vi "Response - Set Status Code.vi"() -> (3 "Unit Test Framework Results":T1)   [LabVIEW 2023, in "Response.lvclass"]
doc: "Use this template to create a user-defined test VI. Define your test requirements and wire the results to the <b>Result (Test)</b> control. Do not modify the <b>Unit Test Framework Results</b> indicator."
uses:
  Response.lvclass
  <vilib>/utf/common/utf_test_comparison_operators.ctl
  <vilib>/utf/NI_UnitTestFramework.lvlib
  <vilib>/utf/common/utf_test_result.ctl
  <vilib>/utf/common/utf_test_result_failure.ctl
  <vilib>/utf/common/utf_test_result_troll.ctl
  <vilib>/utf/common/utf_vi_tag.ctl
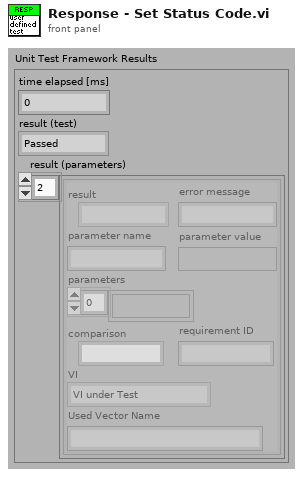
[diagram p1: front panel]
types:
  T1 = typedef "NI_UnitTestFramework.lvlib/utf_test_result_troll.ctl" = cluster{"time elapsed [ms]":u32, "result (test)":T2, "result (parameters)":T3[]}
  T2 = typedef "NI_UnitTestFramework.lvlib/utf_test_result.ctl" = enum16{"Passed", "Failed", "Error", "Skipped", "Not Processed"}
  T3 = typedef "NI_UnitTestFramework.lvlib/utf_test_result_failure.ctl" = cluster{"result":T2, "error message":string, "parameter name":string, "parameter value":variant, "parameters":variant[], "comparison":T4, "requirement ID":string, "VI":T5, "Used Vector Name":string}
  T4 = typedef "NI_UnitTestFramework.lvlib/utf_test_comparison_operators.ctl" = enum16{"=", "!=", ">", ">=", "<", "<=", "range", "symmetric tolerance", "asymmetric tolerance", "string contains", "string not contain", "array size", "string length", "array range", "by element", "array range (limit array)", "user-defined", "array contains", "array not contain", "vector length", "= (elm)", "!= (elm)", "= (case insensitive)", "!= (case insensitive)"}
  T5 = typedef "NI_UnitTestFramework.lvlib/utf_vi_tag.ctl" = enum16{"Setup VI", "VI under Test", "Teardown VI"}
  T6 = typedef "Response.lvclass/Standard Response Messages.ctl" = u16
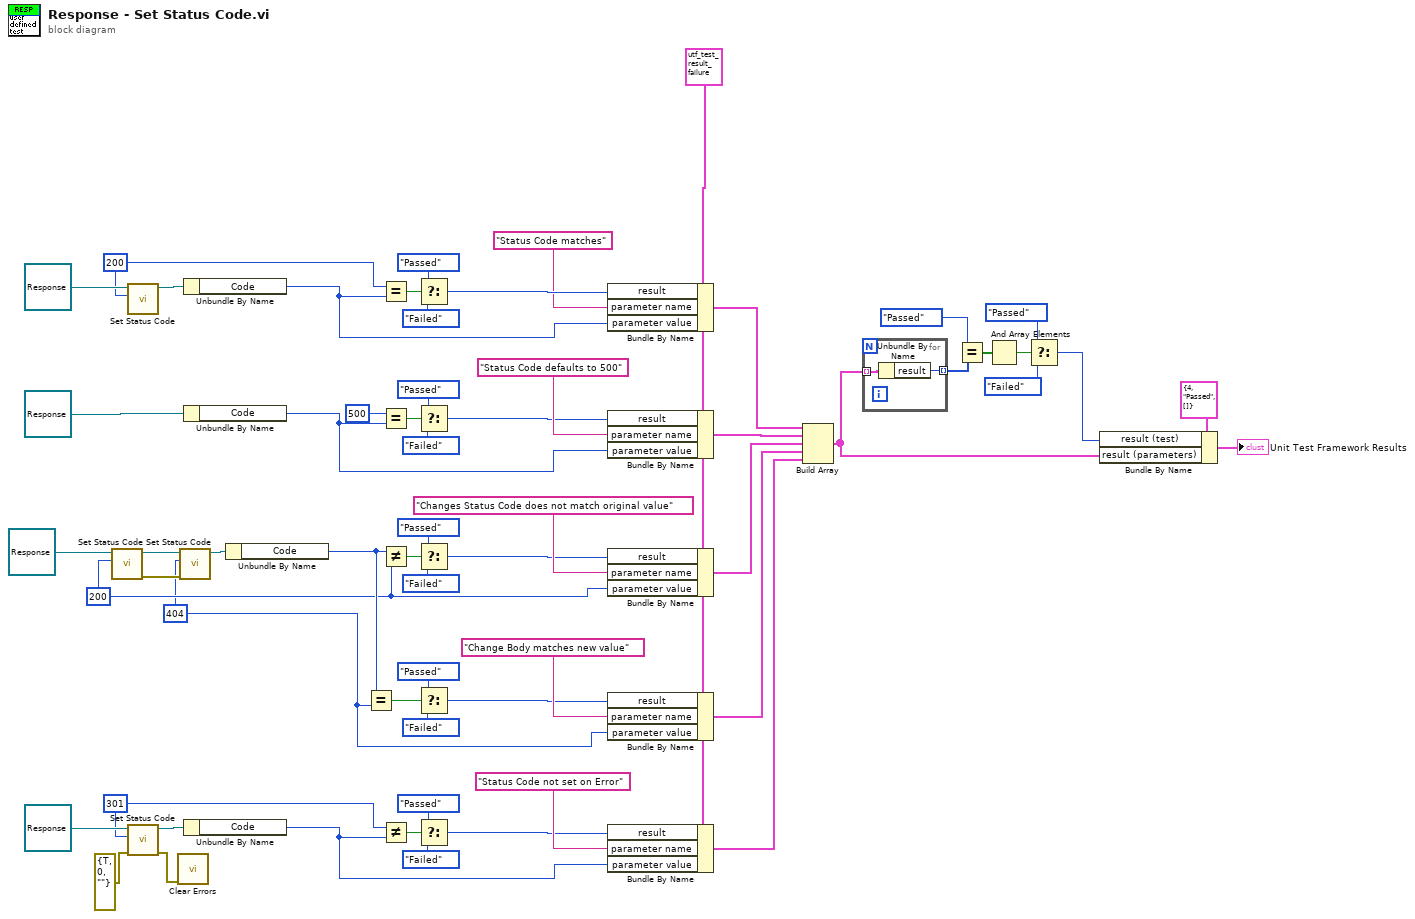
[diagram p0: block diagram]
diagram:
  w5 = u16 301 ("parameter name")
  w3 = u16 404 ("parameter name")
  w4 = u16 200 ("parameter name")
  w2 = u16 200 ("parameter name")
  w9 = T3 {"result"=enum."Not Processed", "error message"="", "parameter name"="", "parameter value"=variant, "parameters"=[], "comparison"=enum."=", "requirement ID"="", "VI"=enum."VI under Test", "Used Vector Name"=""} ("Unit Test Framework - result (parameters)")
  n1 = call "Set Status Code.vi"("Status Code"=w4, "Response in"=refnum<class "Response.lvclass"> refnum) -> ("error out"=w44:errorcluster, "Response out"=w38:refnum<class "Response.lvclass">)  [unwired: 8 in]
  n2 = call "Set Status Code.vi"("Status Code"=w2, "Response in"=refnum<class "Response.lvclass"> refnum) -> ("Response out"=w30:refnum<class "Response.lvclass">)  [unwired: 8 in, 1 out]
  n3 = call "Set Status Code.vi"("error in (no error)"=errorcluster {"status"=TRUE, "code"=0, "source"=""}, "Status Code"=w5, "Response in"=refnum<class "Response.lvclass"> refnum) -> ("error out"=w6:errorcluster, "Response out"=w16:refnum<class "Response.lvclass">)  [unwired: 7 in]
  n4 = call <vilib>:"Clear Errors.vi"("error in (no error)"=w6) -> ()  [unwired: 5 in, 2 out]
  n5 = call "Set Status Code.vi"("error in (no error)"=w44, "Status Code"=w3, "Response in"=w38) -> ("Response out"=w19:refnum<class "Response.lvclass">)  [unwired: 7 in, 1 out]
  n6 = Unbundle By Name(w30) -> ("Code"=w21:T6)
  n7 = Unbundle By Name(refnum<class "Response.lvclass"> refnum ("Response in")) -> ("Code"=w22:T6)
  n8 = Unbundle By Name(w16) -> ("Code"=w17:T6)
  n9 = Unbundle By Name(w19) -> ("Code"=w18:T6)
  n10 = Equal?(x=w18, y=w3) -> (x = y?=w36:bool)
  n11 = Equal?(x=w2, y=w21) -> (x = y?=w48:bool)
  n12 = Equal?(x=u16 500, y=w22) -> (x = y?=w27:bool)
  n13 = Not Equal?(x=w18, y=w4) -> (x != y?=w42:bool)
  n14 = Not Equal?(x=w5, y=w17) -> (x != y?=w13:bool)
  n15 = Select(t=utf_test_result."Passed" ("result"), s=w48, f=utf_test_result."Failed" ("result")) -> (s? t:f=w49:T2)
  n16 = Select(t=utf_test_result."Passed" ("result"), s=w27, f=utf_test_result."Failed" ("result")) -> (s? t:f=w26:T2)
  n17 = Select(t=utf_test_result."Passed" ("result"), s=w42, f=utf_test_result."Failed" ("result")) -> (s? t:f=w41:T2)
  n18 = Select(t=utf_test_result."Passed" ("result"), s=w36, f=utf_test_result."Failed" ("result")) -> (s? t:f=w34:T2)
  n19 = Select(t=utf_test_result."Passed" ("result"), s=w13, f=utf_test_result."Failed" ("result")) -> (s? t:f=w12:T2)
  n20 = Bundle By Name(cluster=w9, "result"=w49, "parameter name"="Status Code matches", "parameter value"=w21) -> (w29:T3)
  n21 = Bundle By Name(cluster=w9, "result"=w26, "parameter name"="Status Code defaults to 500", "parameter value"=w22) -> (w20:T3)
  n22 = Bundle By Name(cluster=w9, "result"=w41, "parameter name"="Changes Status Code does not match original value", "parameter value"=w4) -> (w37:T3)
  n23 = Bundle By Name(cluster=w9, "result"=w34, "parameter name"="Change Body matches new value", "parameter value"=w3) -> (w31:T3)
  n24 = Bundle By Name(cluster=w9, "result"=w12, "parameter name"="Status Code not set on Error", "parameter value"=w17) -> (w8:T3)
  n25 = Build Array(w29, w20, w37, w31, w8) -> (w59:T3[])
  n26 = for {
    tunnel: w59 -> [w63] mode=indexing
    tunnel: [w62] -> w58 mode=indexing
    n27 = Unbundle By Name(w63) -> ("result"=w62:T2)
  }
  n28 = Equal?(x=utf_test_result."Passed" ("result"), y=w58) -> (x = y?=w56:bool[])
  n29 = And Array Elements(Boolean array=w56) -> (logical AND=w55:bool)
  n30 = Select(t=utf_test_result."Passed" ("result"), s=w55, f=utf_test_result."Failed" ("result")) -> (s? t:f=w52:T2)
  n31 = Bundle By Name(cluster=T1 {"time elapsed [ms]"=4, "result (test)"=enum."Passed", "result (parameters)"=[]} ("Unit Test Framework - Result"), "result (test)"=w52, "result (parameters)"=w59) -> (→"Unit Test Framework Results":T1)
